vi "SubPanelVI.vi"() -> ()   [LabVIEW 2012, in "SubPanelsLib.lvlib"]
uses:
  SubPanelsLib.lvlib
panel:
  in  "Sub Panel VI Running":refnum<vi>
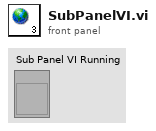
[diagram p1: front panel]
diagram:
